vi "aes_ECU Event Filter.vi"(9 "Cycles to Filter":u16, 10 "Input Signal":bool, 11 "Input Angle (degrees)":fxp<+,61,10>) -> (2 "Output Filtered Signal":bool, 3 "Transitioned Angle":fxp<+,61,10> format="%.55g")   [LabVIEW 2010, in "AES.lvlib" / "AES FPGA.lvlib"]
doc: "This IP is a generic filter that will filter out any noise that occurs less than the number of \"cycles to filter\" that is specified. If it is in fact a digital edge transition whose pulse width is longer than the cycles to filter, the angle where the digital edge occurred is latched out."
uses:
  AES FPGA.lvlib
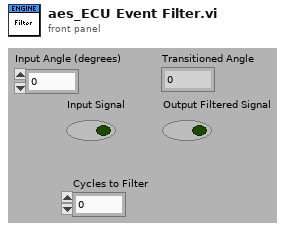
[diagram p1: front panel]
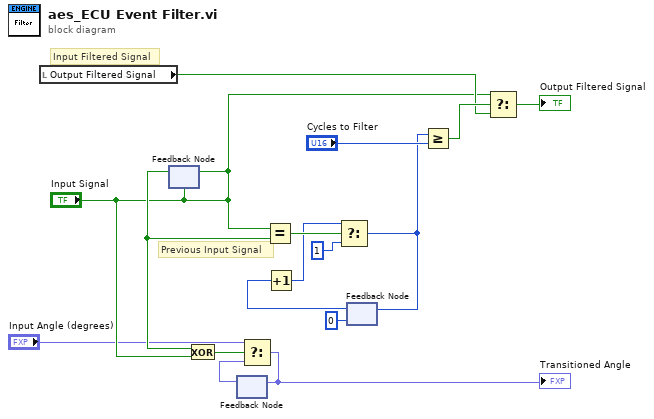
[diagram p0: block diagram]
diagram:
  # "Input Filtered Signal"
  # "Previous Input Signal"
  n1 = local read "Output Filtered Signal"() -> (w10:bool)
  n2 = feedback-in #1("Input Signal") -> ()
  n3 = feedback #1("Input Signal") -> (w6:bool)
  n4 = Exclusive Or(1:"Input Signal", 2:w6) -> (0:w4:bool)
  n5 = feedback #2() -> (w1:fxp<+,61,10>)  [unwired: 1 out]
  n6 = Select(t="Input Angle (degrees)", s=w4, f=w1) -> (s? t:f=w2:fxp<+,61,10>)
  "Transitioned Angle" <- w2
  n7 = feedback-in #2(w2) -> ()
  n8 = Equal?(x="Input Signal", y=w6) -> (x = y?=w15:bool)
  n9 = feedback #3(u16 0 ("f")) -> (w8:u16)
  n10 = Increment(x=w8) -> (x+1=w14:u16)
  n11 = Select(t=w14, s=w15, f=u16 1) -> (s? t:f=w9:u16)
  n12 = feedback-in #3(w9) -> ()
  n13 = Greater Or Equal?(x=w9, y="Cycles to Filter") -> (x >= y?=w11:bool)
  n14 = Select(t="Input Signal", s=w11, f=w10) -> (s? t:f=→"Output Filtered Signal":bool)
